vi "Configure Blanking.vi"(8 "error in (no error)":errorcluster, 10 "Enable Blanking (True)":bool=TRUE, 11 "VISA resource name":refnum<visa-resource-name>) -> (0 "error out":errorcluster, 3 "VISA resource name out":refnum<visa-resource-name>)   [LabVIEW 2015, in "Voltech PM1000+.lvlib"]
doc: "Enables or disables blanking.\n\nNormally Enabled, select Disable to measure voltage or current that is small (<0.25V or <3mA). If blanking operates on either voltage or current then all related measurements will be blanked including W, VA and PF."
uses:
  <instrlib>/Voltech PM1000+/Voltech PM1000+.lvlib
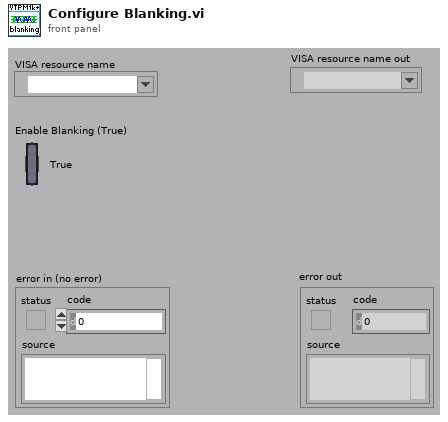
[diagram p1: front panel]
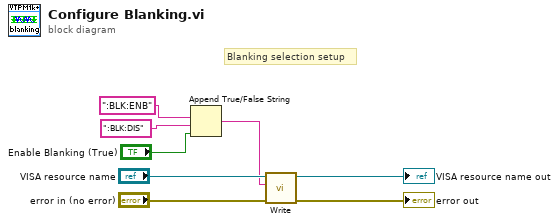
[diagram p0: block diagram]
diagram:
  # "Blanking selection setup"
  n1 = Append True/False String(1:"Enable Blanking (True)", 2:":BLK:DIS", 3:":BLK:ENB") -> (0:w3:string)  [unwired: 1 in]
  n2 = call <instrlib>:"Write.vi"("error in (no error)"="error in (no error)", "Write Buffer"=w3, "VISA resource name"="VISA resource name") -> ("error out"=→"error out":errorcluster, "VISA resource name out"=→"VISA resource name out":refnum<visa-resource-name>)  [unwired: 7 in]
